vi "RelayControlPlottingSBE37andRTD.vi"() -> ()   [LabVIEW 2023]
uses:
  <vilib>/picture/cartesn2.llb/XY Plot Type.ctl
  3107c4ef-b790-5349-8479-afe5556ad064.vi
  <vilib>/Utility/error.llb/Trim Whitespace One-Sided.vi
  <vilib>/Array/Sort 2D Array - Pop Stack.vi
  <vilib>/Array/Sort 2D Array - Push Stack.vi
  <vilib>/Utility/file.llb/Read Delimited Spreadsheet (string).vi
  <vilib>/Utility/file.llb/Write Delimited Spreadsheet (string).vi
  <vilib>/Instr/_visa.llb/VISA Configure Serial Port (Instr).vi
panel:
  in  "autotuning parameters 2":T1={"controller type"=1, "relay cycles"=3, "relay amplitude"=1.0, "control specification"=2, "PV noise level"=0.1} {"PV noise level" format="%.2f"; "control specification" items=["normal", "fast", "slow"]; "relay amplitude" format="%.2f"; "controller type" items=["PID", "PI", "P"]}
  in  "reinitialize? (F)":bool
  out "output":dbl format="%.2f"
  in  "PID gains":T2={"proportional gain (Kc)"=1.0, "integral time (Ti, min)"=0.01, "derivative time (Td, min)"=0.0} {"derivative time (Td, min)" format="%.3f"; "integral time (Ti, min)" format="%.3f"; "proportional gain (Kc)" format="%.3f"}
  in  "setpoint":dbl format="%.2f"
  in  "XY plot cosmetics":T4={"plot color"=16776960, "XY plot type"=enum."connected points", "baseline"=0.0} {"baseline" format="%0.2f"}
  in  "cartesian axis attributes":T5={"x minimum"=0.0, "x maximum"=0.0, "x log?"=FALSE, "x precision"=1, "x format"=enum."Decimal", "y minimum"=0.0, "y maximum"=0.0, "y log?"=FALSE, "y precision"=1, "y format"=enum."Decimal"} {"x minimum" format="%0.2f"; "x maximum" format="%0.2f"; "y minimum" format="%0.2f"; "y maximum" format="%0.2f"}
  out "Table Control 2":string[][](table)
  out "2D Picture 3":picture
  out "Thermometer":dbl(slide) scale=0.0..100.0
  in  "stop":bool
  in  "format (%s)":string="%s"
  out "error out":errorcluster
  in  "VISA resource name 2":refnum<visa-resource-name>
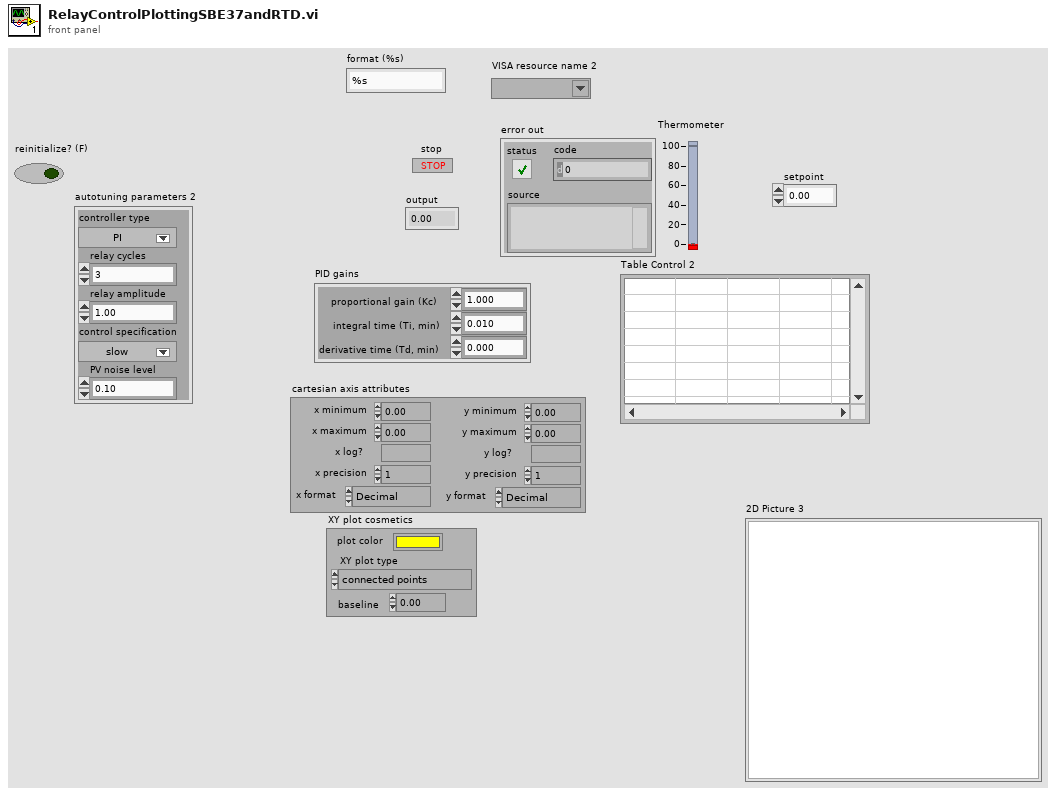
[diagram p1: front panel]
types:
  T1 = cluster{"controller type":u16, "relay cycles":i32, "relay amplitude":dbl, "control specification":u16, "PV noise level":dbl}
  T2 = cluster{"proportional gain (Kc)":dbl, "integral time (Ti, min)":dbl, "derivative time (Td, min)":dbl}
  T3 = typedef "XY Plot Type.ctl" = enum16{"points", "squares", "circles", "connected points", "connected squares", "connected circles", "comb plot", "sized scatter plot", "sized-colored scatter plot", "min-max lines"}
  T4 = cluster{"plot color":u32, "XY plot type":T3, "baseline":dbl}
  T5 = cluster{"x minimum":dbl, "x maximum":dbl, "x log?":bool, "x precision":u8, "x format":enum8{"Decimal", "Scientific", "Engineering", "Binary", "Octal", "Hex"}, "y minimum":dbl, "y maximum":dbl, "y log?":bool, "y precision":u8, "y format":enum8{"Decimal", "Scientific", "Engineering", "Binary", "Octal", "Hex"}}
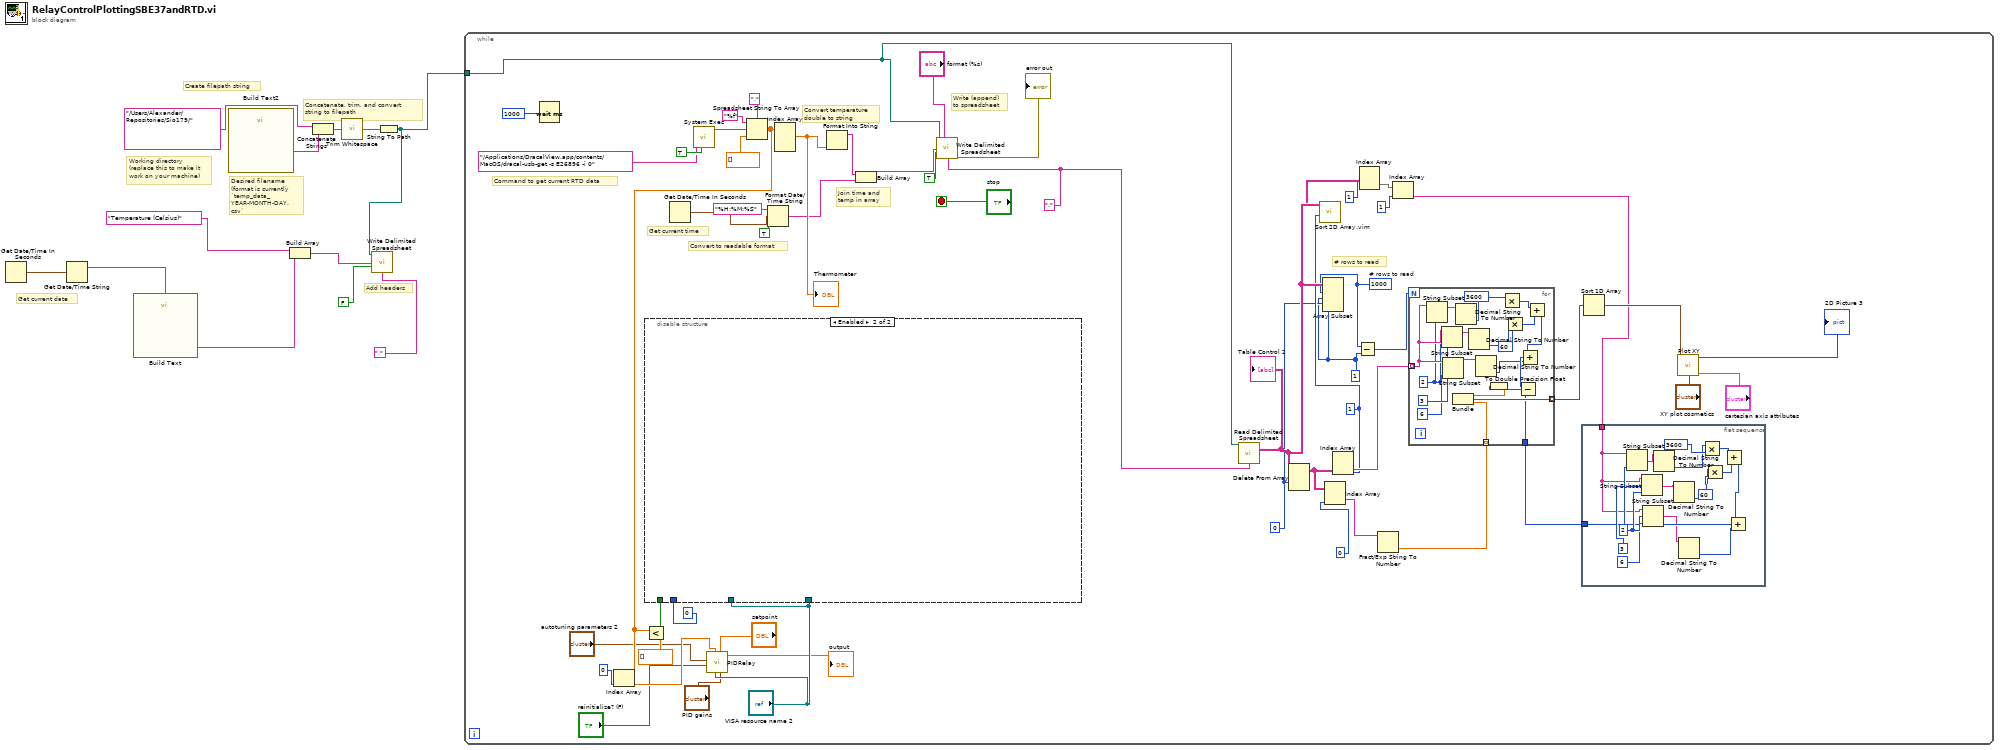
[diagram p0: block diagram]
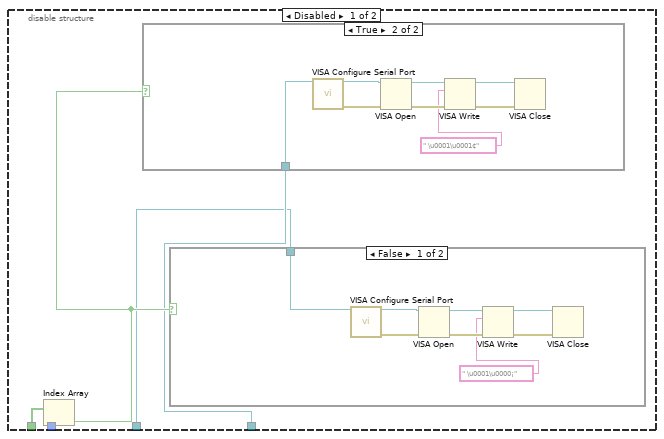
[diagram p2: hidden frame]
diagram:
  # "Add headers"
  # "Get current date"
  # "Concatenate, trim, and convert string to filepath"
  # "Desired filename (format is currently `temp_data_YEAR-MONTH-DAY.csv`"
  # "Working directory (replace this to make it work on your machine)"
  # "Create filepath string"
  n1 = Get Date/Time In Seconds() -> (seconds since 1Jan1904=w10:timestamp)
  n2 = Get Date/Time String(seconds (now)=w10) -> (date string=w6:string)  [unwired: 2 in, 1 out]
  n3 = call "Build Text"("date"=w6) -> ("Result"=w9:string)  [unwired: 13 in, 1 out]
  n4 = call "Build Text2"() -> ("Result"=w5:string)  [unwired: 14 in, 1 out]
  n5 = Build Array("Temperature (Celsius)", w9) -> (w8:string[])
  n6 = Concatenate Strings("/Users/Alexander/Repositories/Sio179/", w5) -> (w11:string)
  n7 = call <vilib>:"Trim Whitespace.vi"("string"=w11) -> ("trimmed string"=w12:string)  [unwired: 1 in]
  n8 = String To Path(string=w12) -> (path=w7:path)
  n9 = call-poly <vilib>:"Write Delimited Spreadsheet.vi"("file path (dialog if empty)"=w7, "1D data"=w8, "append to file? (new file:F)"=FALSE, "delimiter (\\t)"=",") -> ()  [unwired: 10 in, 2 out]
  n10 = while {
    tunnel: w7 -> [w36]
    stop <- "stop" stop-if-true
    w26 = ","
    w35 = 1000  # # rows to read
    w38 = 1
    w40 = 1
    w39 = 0
    # "# rows to read"
    # "Command to get current RTD data"
    # "Join time and temp in array"
    # "Convert temperature double to string"
    # "Convert to readable format"
    # "Get current time"
    # "Write (append) to spreadsheet"
    n11 = Wait (ms)(milliseconds to wait=u32 1000 ("millisecond timer value")) -> ()  [unwired: 1 out]
    n12 = Get Date/Time In Seconds() -> (seconds since 1Jan1904=w31:timestamp)
    n13 = call <vilib>:"System Exec.vi"("run minimized? (F)"=TRUE, "command line"="/Applications/DracalView.app/contents/MacOS/dracal-usb-get -s E26896 -i 0") -> ("standard output"=w62:string)  [unwired: 6 in, 3 out]
    n14 = Spreadsheet String To Array(delimiter (Tab)=",", format string="%f", spreadsheet string=w62, array type (2D Dbl)=dbl[] [] ("Array")) -> (array=w21:dbl[])
    n15 = Index Array(array=w21, index=0) -> (element=w20:dbl)
    n16 = Less?(x=w21, y=dbl[] []) -> (x < y?=w54:bool[])
    n17 = disable-structure shown="Enabled" {
      disable-tunnel: w54 -> [w70 _]
      disable-tunnel: 0 ("index") -> [w69 _]
      disable-tunnel: "VISA resource name 2" -> [w68 _]
      disable-tunnel: "VISA resource name 2" -> [w67 _]
      frame Disabled {
        n18 = Index Array(array=w70, index=w69) -> (element=w71:bool)
        n19 = case shown="True" w71 {
          tunnel: w68 -> [_ w80]
          frame False {
          }
          frame True {
            n20 = call-poly "VISA Configure Serial Port"("VISA resource name"=w80) -> ("VISA resource name out"=w87:refnum<visa-resource-name>, "error out"=w86:errorcluster)  [unwired: 13 in]
            n21 = VISA Open(error in (no error)=w86, VISA resource name=w87) -> (VISA resource name=w85:refnum<visa-resource-name>, error out=w84:errorcluster)  [unwired: 3 in]
            n22 = VISA Write(VISA resource name=w85, write buffer=" \u0001\u0001¢", error in (no error)=w84) -> (VISA resource name out=w83:refnum<visa-resource-name>, error out=w82:errorcluster)  [unwired: 1 out]
            n23 = VISA Close(VISA resource name=w83, error in (no error)=w82) -> ()  [unwired: 1 out]
          }
        }
        n24 = case shown="False" w71 {
          tunnel: w67 -> [w72 _]
          frame False {
            n25 = call-poly "VISA Configure Serial Port"("VISA resource name"=w72) -> ("VISA resource name out"=w79:refnum<visa-resource-name>, "error out"=w78:errorcluster)  [unwired: 13 in]
            n26 = VISA Open(error in (no error)=w78, VISA resource name=w79) -> (VISA resource name=w77:refnum<visa-resource-name>, error out=w76:errorcluster)  [unwired: 3 in]
            n27 = VISA Write(VISA resource name=w77, write buffer=" \u0001\u0000¡", error in (no error)=w76) -> (VISA resource name out=w75:refnum<visa-resource-name>, error out=w74:errorcluster)  [unwired: 1 out]
            n28 = VISA Close(VISA resource name=w75, error in (no error)=w74) -> ()  [unwired: 1 out]
          }
          frame True {
          }
        }
      }
      frame Enabled {
      }
    }
    n29 = call "PIDRelay.vi"("PID gains"="PID gains", "setpoint"="setpoint", "VISA resource name 2"="VISA resource name 2", "process variable"=w20, "reinitialize? (F)"="reinitialize? (F)", "autotuning parameters 2"="autotuning parameters 2") -> ("output"=→"output":dbl)  [unwired: 5 in]
    n30 = Format Date/Time String(time format string (%c)="%H:%M:%S", seconds (now)=w31, UTC format=TRUE) -> (date/time string=w34:string)
    n31 = Index Array(array=w21) -> (element #1=w52:dbl)  [unwired: 3 in, 2 out]
    "Thermometer" <- w52
    n32 = Format Into String(w52) -> (resulting string=w55:string)  [unwired: 3 in, 1 out]
    n33 = Build Array(w55, w34) -> (w56:string[])
    n34 = call-poly <vilib>:"Write Delimited Spreadsheet.vi"("file path (dialog if empty)"=w36, "format (%s)"="format (%s)", "1D data"=w56, "append to file? (new file:F)"=TRUE, "delimiter (\\t)"=w26) -> ("error out"=→"error out":errorcluster)  [unwired: 9 in, 1 out]
    n35 = call-poly <vilib>:"Read Delimited Spreadsheet.vi"("file path (dialog if empty)"=w36, "delimiter (\\t)"=w26) -> ("all rows"=w42:string[][])  [unwired: 8 in, 5 out]
    "Table Control 2" <- w42
    n36 = Delete From Array(array=w42, index (row)=w39) -> (array with subset deleted=w51:string[][])  [unwired: 2 in, 1 out]
    n37 = call "Sort 2D Array.vim"("index"=w40, "2D array"=w42) -> ("sorted 2D array"=w41:string[][])  [unwired: 8 in, 1 out]
    n38 = Array Subset(array=w42, index (row)=w35, length (row)=w38, index (col)=w39, length (col)=w38) -> ()  [unwired: 1 out]
    n39 = Index Array(array=w51, index (col)=0) -> (element=w30:string[])  [unwired: 1 in]
    n40 = Index Array(array=w51, index (col)=w40) -> (element=w49:string[])  [unwired: 1 in]
    n41 = Subtract(x=w35, y=w38) -> (x-y=w50:i32)
    n42 = Index Array(array=w41, index (row)=1) -> (element=w44:string[])  [unwired: 1 in]
    n43 = Fract/Exp String To Number(string=w30) -> (number=w29:dbl[])  [unwired: 3 in, 1 out]
    n44 = Index Array(array=w44, index=1) -> (element=w43:string)
    n45 = for {
      N: w50 -> [_]
      tunnel: w49 -> [w122] mode=indexing
      tunnel: [w124] -> w47 mode=indexing
      tunnel: w45 -> [w111]
      tunnel: w29 -> [w104] mode=indexing
      w121 = 2
      n46 = String Subset(string=w122, length (rest)=w121) -> (substring=w105:string)  [unwired: 1 in]
      n47 = String Subset(string=w122, offset (0)=3, length (rest)=w121) -> (substring=w108:string)
      n48 = String Subset(string=w122, offset (0)=6, length (rest)=w121) -> (substring=w109:string)
      n49 = Decimal String To Number(string=w105) -> (number=w106:i32)  [unwired: 2 in, 1 out]
      n50 = Decimal String To Number(string=w108) -> (number=w107:i32)  [unwired: 2 in, 1 out]
      n51 = Decimal String To Number(string=w109) -> (number=w110:i32)  [unwired: 2 in, 1 out]
      n52 = Multiply(x=w106, y=3600) -> (x*y=w116:i32)
      n53 = Multiply(x=w107, y=60) -> (x*y=w115:i32)
      n54 = Add(x=w116, y=w115) -> (x+y=w114:i32)
      n55 = Add(x=w114, y=w110) -> (x+y=w113:i32)
      n56 = Subtract(x=w113, y=w111) -> (x-y=w112:i32)
      n57 = To Double Precision Float(number=w112) -> (double precision float=w123:dbl)
      n58 = Bundle(w123, "String"=w104) -> (w124:cluster{dbl, "String":dbl})  [unwired: 1 in]
    }
    n59 = flat-sequence {
      tunnel: [w95] -> w45
      tunnel: w43 -> [w94]
      frame #0 {
        w98 = 2
        n60 = String Subset(string=w94, length (rest)=w98) -> (substring=w91:string)  [unwired: 1 in]
        n61 = String Subset(string=w94, offset (0)=3, length (rest)=w98) -> (substring=w92:string)
        n62 = String Subset(string=w94, offset (0)=6, length (rest)=w98) -> (substring=w93:string)
        n63 = Decimal String To Number(string=w91) -> (number=w90:i32)  [unwired: 2 in, 1 out]
        n64 = Decimal String To Number(string=w92) -> (number=w89:i32)  [unwired: 2 in, 1 out]
        n65 = Decimal String To Number(string=w93) -> (number=w88:i32)  [unwired: 2 in, 1 out]
        n66 = Multiply(x=w90, y=3600) -> (x*y=w103:i32)
        n67 = Multiply(x=w89, y=60) -> (x*y=w102:i32)
        n68 = Add(x=w103, y=w102) -> (x+y=w101:i32)
        n69 = Add(x=w101, y=w88) -> (x+y=w95:i32)
      }
    }
    n70 = Sort 1D Array(array=w47) -> (sorted array=w46:cluster{dbl, "String":dbl}[])
    n71 = call <vilib>:"Plot XY.vi"("data"=w46, "cartesian axis attributes"="cartesian axis attributes", "XY plot cosmetics"="XY plot cosmetics") -> ("new picture"=→"2D Picture 3":picture)  [unwired: 12 in]
  }
